vi "test_plugin.vi"(7 "LabVIEW Web Service Request":refnum<class "Web Request.lvclass">, 11 "context_id":string) -> (2 "g4l_api_version":string, 3 "valid":bool)   [LabVIEW 2013]
uses:
  <vilib>/wsapi/Web Request.lvclass
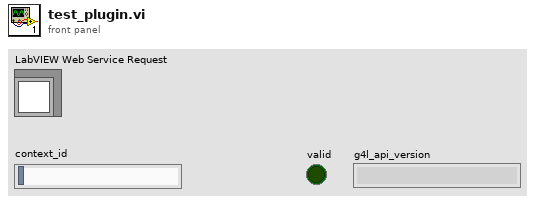
[diagram p1: front panel]
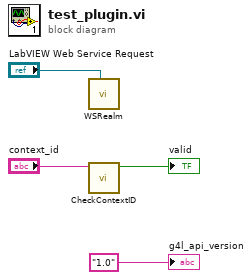
[diagram p0: block diagram]
diagram:
  n1 = call "WSRealm.vi"("LabVIEW Web Service Request"="LabVIEW Web Service Request") -> ()  [unwired: 11 in]
  n2 = call "CheckContextID.vi"("context_id"="context_id") -> ("valid"=→"valid":bool)  [unwired: 10 in]
  "g4l_api_version" <- "1.0"
